vi "Read Dashboard Variables.vi"() -> ()   [LabVIEW 2020]
uses:
  <vilib>/Rock Robotics/Network Tables/NT Read Number.vi
  Robot Global Data.vi
panel:
  out "Limelight tv":dbl format="%_6g"
  out "Limelight ta":dbl format="%_6g"
  out "Limelight tx":dbl format="%_6g"
  out "MaxDrive":dbl(slide)=0.6824817518248175 min=0.0 max=1.0 step=0.01 scale=0.0..1.0
  out "DriveK":dbl(slide)=0.26277372262773724 min=0.0 max=1.0 step=0.05 scale=0.0..1.0
  out "Limelight Goal Area":dbl(slide)=14.872262773722628 min=0.1 max=25.0 step=0.25 scale=0.0..25.0
  out "AimDeadband":dbl min=0.0 max=10.0 step=0.25
  out "MinSteerCommand":dbl(slide)=0.2717391304347826 min=0.0 max=0.5 step=0.05 scale=0.0..0.5
  out "SteeringK":dbl(slide)=0.025362318840579712 min=0.0 max=0.25 step=0.01 scale=0.0..0.25
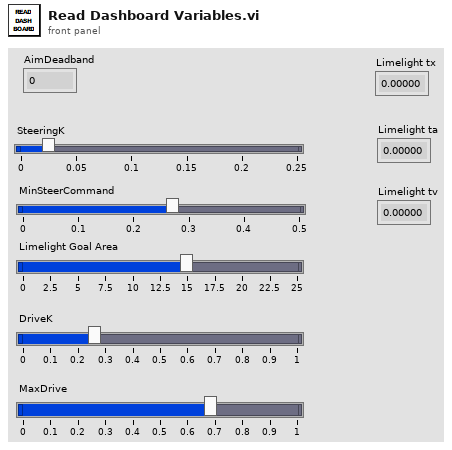
[diagram p1: front panel]
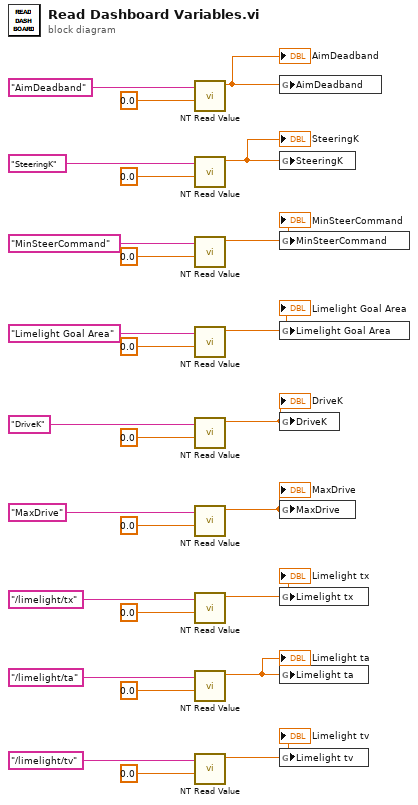
[diagram p0: block diagram]
diagram:
  n1 = call-poly <vilib>:"NT Read Value.vi"("Default Value"=0.0, "Name"="AimDeadband") -> ("Numeric"=w25:dbl)  [unwired: 8 in, 1 out]
  "AimDeadband" <- w25
  n2 = call-poly <vilib>:"NT Read Value.vi"("Default Value"=0.0, "Name"="SteeringK") -> ("Numeric"=w8:dbl)  [unwired: 8 in, 1 out]
  "SteeringK" <- w8
  n3 = call-poly <vilib>:"NT Read Value.vi"("Default Value"=0.0, "Name"="MinSteerCommand") -> ("Numeric"=w7:dbl)  [unwired: 8 in, 1 out]
  "MinSteerCommand" <- w7
  n4 = call-poly <vilib>:"NT Read Value.vi"("Default Value"=0.0, "Name"="Limelight Goal Area") -> ("Numeric"=w6:dbl)  [unwired: 8 in, 1 out]
  "Limelight Goal Area" <- w6
  n5 = call-poly <vilib>:"NT Read Value.vi"("Default Value"=0.0, "Name"="DriveK") -> ("Numeric"=w5:dbl)  [unwired: 8 in, 1 out]
  "DriveK" <- w5
  n6 = call-poly <vilib>:"NT Read Value.vi"("Default Value"=0.0, "Name"="MaxDrive") -> ("Numeric"=w4:dbl)  [unwired: 8 in, 1 out]
  "MaxDrive" <- w4
  n7 = call-poly <vilib>:"NT Read Value.vi"("Default Value"=0.0, "Name"="/limelight/tx") -> ("Numeric"=w3:dbl)  [unwired: 8 in, 1 out]
  "Limelight tx" <- w3
  n8 = call-poly <vilib>:"NT Read Value.vi"("Default Value"=0.0, "Name"="/limelight/ta") -> ("Numeric"=w2:dbl)  [unwired: 8 in, 1 out]
  "Limelight ta" <- w2
  n9 = call-poly <vilib>:"NT Read Value.vi"("Default Value"=0.0, "Name"="/limelight/tv") -> ("Numeric"=w1:dbl)  [unwired: 8 in, 1 out]
  "Limelight tv" <- w1
  n10 = global write "Robot Global Data.vi" "AimDeadband"(w25) -> ()
  n11 = global write "Robot Global Data.vi" "SteeringK"(w8) -> ()
  n12 = global write "Robot Global Data.vi" "MinSteerCommand"(w7) -> ()
  n13 = global write "Robot Global Data.vi" "Limelight Goal Area"(w6) -> ()
  n14 = global write "Robot Global Data.vi" "DriveK"(w5) -> ()
  n15 = global write "Robot Global Data.vi" "MaxDrive"(w4) -> ()
  n16 = global write "Robot Global Data.vi" "Limelight tx"(w3) -> ()
  n17 = global write "Robot Global Data.vi" "Limelight ta"(w2) -> ()
  n18 = global write "Robot Global Data.vi" "Limelight tv"(w1) -> ()
